vi "Refresh Add New Signals.vi"(8 "error in":errorcluster, 10 "Signals":T2[](array[typedef]), 11 "Refresh Signals":T1[](array[typedef])) -> (0 "error out":errorcluster, 3 "Refresh Signals out":T1[](array[typedef]))   [LabVIEW 2020, in "Communication Bus Template System Explorer.lvlib" / "Implementation.lvlib"]
uses:
  Implementation.lvlib
  Types/Refresh Signal.ctl
  Types/Signal.ctl
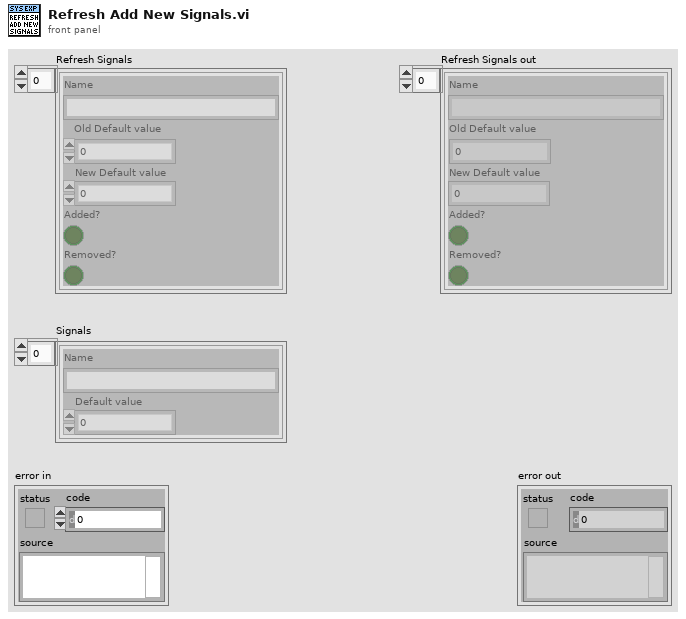
[diagram p1: front panel]
types:
  T1 = typedef "Communication Bus Template System Explorer.lvlib/Implementation.lvlib/Refresh Signal.ctl" = cluster{"Name":string, "Old Default value":dbl, "New Default value":dbl, "Added?":bool, "Removed?":bool}
  T2 = typedef "Communication Bus Template System Explorer.lvlib/Implementation.lvlib/Signal.ctl" = cluster{"Name":string, "Default value":dbl}
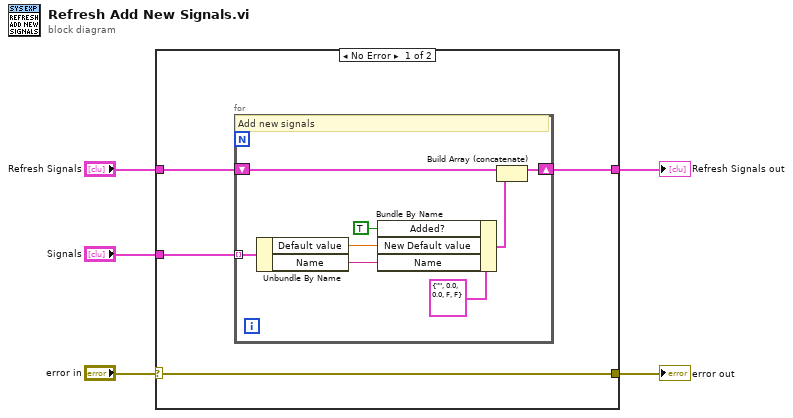
[diagram p0: block diagram]
diagram:
  n1 = case shown="No Error" "error in" {
    selector: "error in" -> [w9 w19]
    tunnel: [w9 w19] -> w4
    tunnel: "Refresh Signals" -> [w8 w18]
    tunnel: "Signals" -> [w7 _]
    tunnel: [w6 w18] -> w1
    frame No Error {
      n2 = for {
        tunnel: w7 -> [w17] mode=indexing
        shift-right: [w13] -> w6
        shift-left: w8 -> [w14]
        # "Add new signals"
        n3 = Unbundle By Name(w17) -> ("Default value"=w11:dbl, "Name"=w12:string)
        n4 = Bundle By Name(cluster=T1 {"Name"="", "Old Default value"=0.0, "New Default value"=0.0, "Added?"=FALSE, "Removed?"=FALSE} ("Refresh Signal"), "Added?"=TRUE, "New Default value"=w11, "Name"=w12) -> (w16:T1)
        n5 = Build Array (concatenate)(w14, w16) -> (w13:T1[])
      }
    }
    frame Error {
    }
  }
  "error out" <- w4
  "Refresh Signals out" <- w1
